vi "Radial_Averaging_V2.vi"(6 "Radial Resolution [pixel]":dbl=1.0, 9 "Center Position [Pixel]":cluster{"Cursor X":dbl, "Cursor Y":dbl}={"Cursor X"=2.5, "Cursor Y"=2.5}, 10 "Pixel Width [um/pixel]":dbl=1.0 format="%.2f", 11 "Image":dbl[][](graph)=[[973.0, 1008.0, 1063.0, 974.0, 895.0], [1059.0, 1159.0, 1209.0, 1166.0, 1007.0], [1101.0, 1203.0, 1245.0, 1186.0, 1054.0], [1069.0, 1169.0, 1219.0, 1148.0, 1059.0], [978.0, 1111.0, 1126.0, 1087.0, 1007.0]]) -> (0 "Radial Average":dbl[](array[numeric])=[1199.5, 1134.125, 1035.9166666666667, 973.0] format="%.2f", 1 "Radius [um]":dbl[](array[numeric])=[0.0, 1.0, 2.0, 3.0] format="%.2f", 2 "Y-Average":dbl[](array[numeric]), 3 "X-Average":dbl[](array[numeric]))   [LabVIEW 2010]
panel:
  out "Radial Average Plot":cluster{dbl[], dbl[]}(graph)={[0.0, 1.0, 2.0, 3.0], [1199.5, 1134.125, 1035.9166666666667, 973.0]}
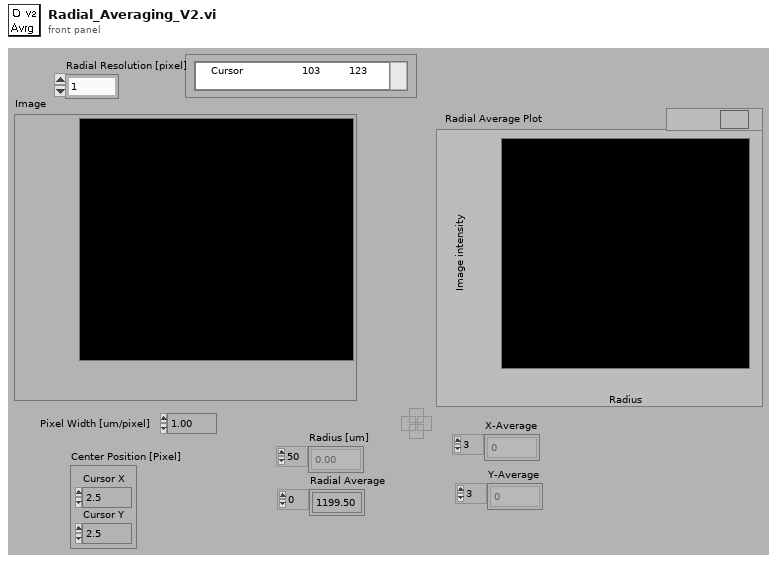
[diagram p1: front panel]
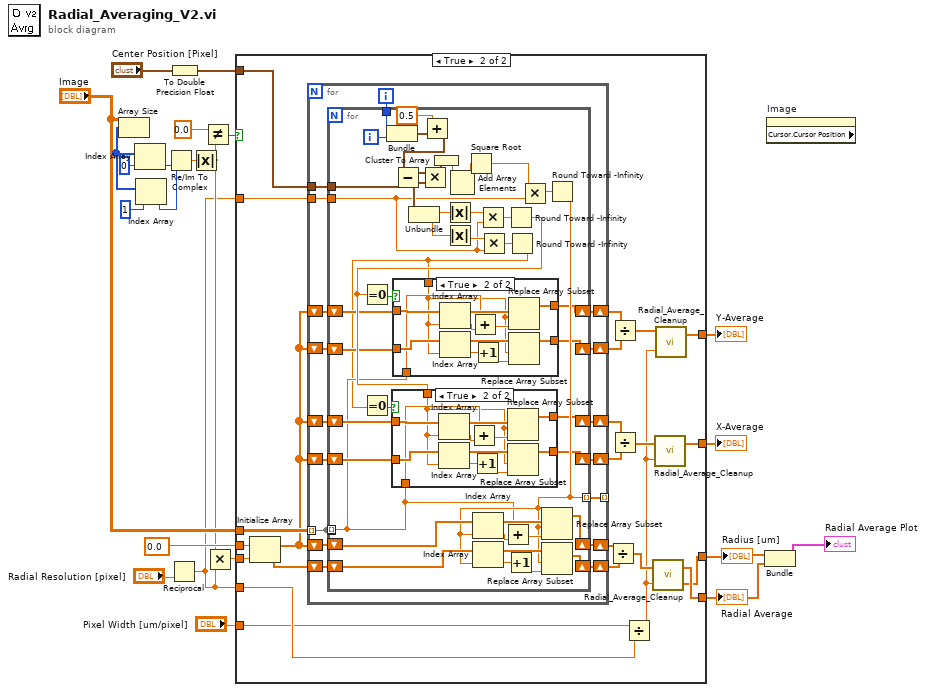
[diagram p0: block diagram]
diagram:
  n1 = Array Size(array="Image") -> (size(s)=w21:i32[])
  n2 = Index Array(array=w21, index=0 ("Index")) -> (element=w18:i32)
  n3 = Index Array(array=w21, index=1 ("Index")) -> (element=w17:i32)
  n4 = Re/Im To Complex(1:w17, 2:w18) -> (0:w16:cdb)
  n5 = Reciprocal(x="Radial Resolution [pixel]") -> (1/x=w5:dbl)
  n6 = To Double Precision Float(number="Center Position [Pixel]") -> (double precision float=w12:cluster{"Cursor X":dbl, "Cursor Y":dbl})
  n7 = Absolute Value(x=w16) -> (abs(x)=w6:dbl)
  n8 = Not Equal?(x=0.0, y=w6) -> (x != y?=w14:bool)
  n9 = Multiply(x=w6, y=w5) -> (x*y=w7:dbl)
  n10 = case shown="True" w14 {
    tunnel: w7 -> [_ w44]
    tunnel: "Image" -> [_ w42]
    tunnel: 0.0 ("y") -> [_ w41]
    tunnel: [_ w40] -> w10
    tunnel: [_ w39] -> w11
    tunnel: w12 -> [_ w38]
    tunnel: w5 -> [_ w37]
    tunnel: w5 -> [_ w34]
    tunnel: "Pixel Width [um/pixel]" -> [_ w33]
    tunnel: [_ w29] -> w3
    tunnel: [_ w23] -> w2
    frame False {
    }
    frame True {
      n11 = Initialize Array(w41, w44) -> (w28:dbl[])
      n12 = for {
        tunnel: w42 -> [w60] mode=indexing
        shift-right: [w59] -> w43
        shift-left: w28 -> [w57]
        shift-right: [w58] -> w35
        shift-left: w28 -> [w56]
        tunnel: w38 -> [w55]
        tunnel: [w54] -> _ mode=indexing
        tunnel: w37 -> [w53]
        shift-right: [w49] -> w32
        shift-left: w28 -> [w52]
        shift-right: [w50] -> w31
        shift-left: w28 -> [w51]
        shift-right: [w46] -> w27
        shift-left: w28 -> [w47]
        shift-right: [w45] -> w26
        shift-left: w28 -> [w48]
        i -> [w61]
        n13 = for {
          tunnel: w60 -> [_] mode=indexing
          tunnel: w61 -> [w94]
          tunnel: w60 -> [w63] mode=indexing
          shift-right: [w102] -> w58
          shift-left: w56 -> [w96]
          shift-right: [w97] -> w59
          shift-left: w57 -> [w95]
          tunnel: w55 -> [w92]
          tunnel: [w86] -> w54 mode=indexing
          tunnel: w53 -> [w75]
          shift-right: [w70] -> w49
          shift-left: w52 -> [w81]
          shift-right: [w71] -> w50
          shift-left: w51 -> [w82]
          shift-right: [w66] -> w46
          shift-left: w47 -> [w65]
          shift-right: [w67] -> w45
          shift-left: w48 -> [w64]
          i -> [w93]
          n14 = Bundle(w94, w93) -> (w91:cluster{i32, i32})  [unwired: 1 in]
          n15 = Add(x=0.5, y=w91) -> (x+y=w90:cluster{dbl, dbl})
          n16 = Subtract(x=w90, y=w92) -> (x-y=w80:cluster{dbl, dbl})
          n17 = Unbundle(w80) -> (w79:dbl, w78:dbl)
          n18 = Multiply(x=w80, y=w80) -> (x*y=w85:cluster{dbl, dbl})
          n19 = Cluster To Array(cluster=w85) -> (array=w84:dbl[])
          n20 = Absolute Value(x=w79) -> (abs(x)=w77:dbl)
          n21 = Absolute Value(x=w78) -> (abs(x)=w76:dbl)
          n22 = Add Array Elements(numeric array=w84) -> (sum=w83:dbl)
          n23 = Square Root(x=w83) -> (sqrt(x)=w88:dbl)
          n24 = Multiply(x=w77, y=w75) -> (x*y=w74:dbl)
          n25 = Multiply(x=w76, y=w75) -> (x*y=w73:dbl)
          n26 = Round Toward -Infinity(1:w74) -> (0:w68:dbl)
          n27 = Equal To 0?(x=w68) -> (x = 0?=w69:bool)
          n28 = Round Toward -Infinity(1:w73) -> (0:w62:dbl)
          n29 = Equal To 0?(x=w62) -> (x = 0?=w72:bool)
          n30 = case shown="True" w72 {
            tunnel: w82 -> [w116 w122]
            tunnel: w81 -> [w115 w121]
            tunnel: w63 -> [_ w120]
            tunnel: w68 -> [_ w119]
            tunnel: [w116 w118] -> w71
            tunnel: [w115 w117] -> w70
            frame False {
            }
            frame True {
              n31 = Index Array(array=w122, index=w119) -> (element=w125:dbl)
              n32 = Index Array(array=w121, index=w119) -> (element=w123:dbl)
              n33 = Add(x=w120, y=w125) -> (x+y=w126:dbl)
              n34 = Increment(x=w123) -> (x+1=w124:dbl)
              n35 = Replace Array Subset(array=w122, new element=w126, index=w119) -> (w118:dbl[])
              n36 = Replace Array Subset(array=w121, new element=w124, index=w119) -> (w117:dbl[])
            }
          }
          n37 = case shown="True" w69 {
            tunnel: w65 -> [w104 w110]
            tunnel: w64 -> [w103 w109]
            tunnel: w63 -> [_ w108]
            tunnel: w62 -> [_ w107]
            tunnel: [w104 w106] -> w66
            tunnel: [w103 w105] -> w67
            frame False {
            }
            frame True {
              n38 = Index Array(array=w110, index=w107) -> (element=w113:dbl)
              n39 = Index Array(array=w109, index=w107) -> (element=w111:dbl)
              n40 = Add(x=w108, y=w113) -> (x+y=w114:dbl)
              n41 = Increment(x=w111) -> (x+1=w112:dbl)
              n42 = Replace Array Subset(array=w110, new element=w114, index=w107) -> (w106:dbl[])
              n43 = Replace Array Subset(array=w109, new element=w112, index=w107) -> (w105:dbl[])
            }
          }
          n44 = Multiply(x=w88, y=w75) -> (x*y=w87:dbl)
          n45 = Round Toward -Infinity(1:w87) -> (0:w86:dbl)
          n46 = Index Array(array=w96, index=w86) -> (element=w99:dbl)
          n47 = Index Array(array=w95, index=w86) -> (element=w101:dbl)
          n48 = Add(x=w63, y=w99) -> (x+y=w98:dbl)
          n49 = Increment(x=w101) -> (x+1=w100:dbl)
          n50 = Replace Array Subset(array=w96, new element=w98, index=w86) -> (w102:dbl[])
          n51 = Replace Array Subset(array=w95, new element=w100, index=w86) -> (w97:dbl[])
        }
      }
      n52 = Divide(x=w35, y=w43) -> (x/y=w36:dbl[])
      n53 = Divide(x=w27, y=w26) -> (x/y=w25:dbl[])
      n54 = Divide(x=w31, y=w32) -> (x/y=w30:dbl[])
      n55 = Divide(x=w33, y=w34) -> (x/y=w24:dbl)
      n56 = call "Radial_Average_Cleanup.vi"("Radial Resolution"=w24, "Averages"=w36) -> ("Radius"=w39:dbl[], "Averages"=w40:dbl[])
      n57 = call "Radial_Average_Cleanup.vi"("Radial Resolution"=w24, "Averages"=w30) -> ("Averages"=w29:dbl[])  [unwired: 1 out]
      n58 = call "Radial_Average_Cleanup.vi"("Radial Resolution"=w24, "Averages"=w25) -> ("Averages"=w23:dbl[])  [unwired: 1 out]
    }
  }
  "Radius [um]" <- w11
  "Radial Average" <- w10
  "X-Average" <- w3
  "Y-Average" <- w2
  n59 = Bundle("Radius"=w11, "Averages"=w10) -> (→"Radial Average Plot":cluster{"Radius":dbl[], "Averages":dbl[]})  [unwired: 1 in]
  n60 = property on="Image" class="IntGraph (strict)" props=["Cursor", "Cursor Position"]() -> ()  [unwired: 2 in, 3 out]
